vi "Parse.vi"(8 "Error In":errorcluster, 11 "Tokens":refnum<class "Abstract.lvclass">[](array[class])) -> (0 "Error Out":errorcluster, 3 "Abstract Syntax Tree":refnum<class "Root.lvclass">)   [LabVIEW 2018, in "Toolkit.lvlib"]
uses:
  Toolkit.lvlib
  Nodes/Root/Root.lvclass
  D:/Users/cfield/Code/Field R&D Services/Mustache/trunk/src/Toolkit/Low-Level/Nodes/NonTerminal/NonTerminal.lvclass
  Tokens/Abstract/Abstract.lvclass
  Nodes/NonTerminal/NonTerminal.lvclass
  D:/Users/cfield/Code/Field R&D Services/Mustache/trunk/src/Toolkit/Low-Level/Nodes/Abstract/Abstract.lvclass
  Tokens/Text/Text.lvclass
  Nodes/Section/Section.lvclass
  Nodes/Tag/Tag.lvclass
  Nodes/Text/Text.lvclass
  Tokens/Text/API/Read Content.vi
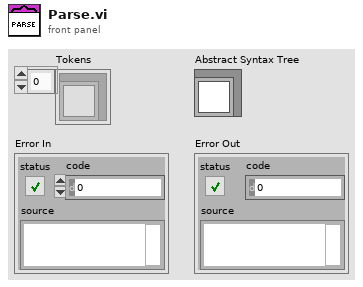
[diagram p1: front panel]
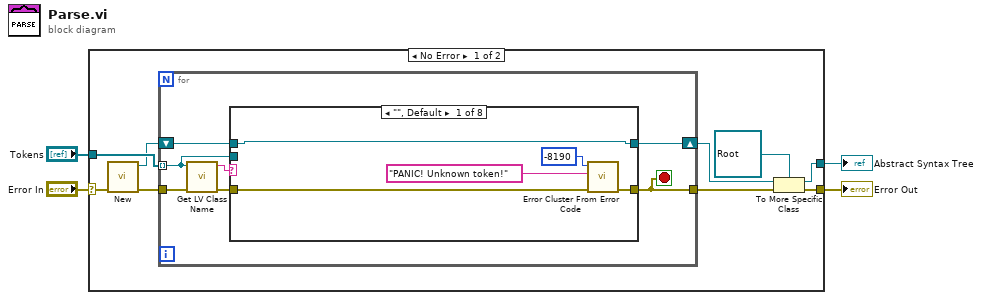
[diagram p0: block diagram]
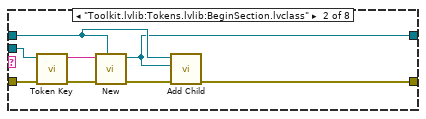
[diagram p2: hidden frame]
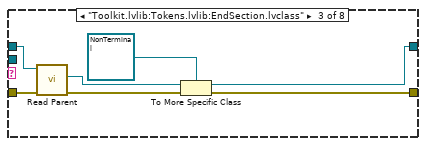
[diagram p3: hidden frame]
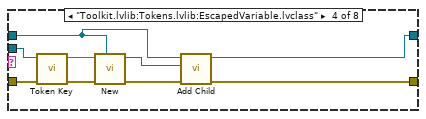
[diagram p4: hidden frame]
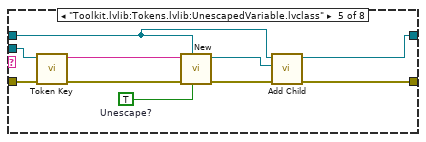
[diagram p5: hidden frame]
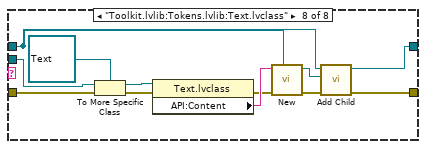
[diagram p8: hidden frame]
diagram:
  n1 = case shown="No Error" "Error In" {
    selector: "Error In" -> [w5 w76]
    tunnel: [w12 w76] -> w3
    tunnel: [w9 _] -> w2
    tunnel: "Tokens" -> [w8 _]
    frame No Error {
      n2 = call "New.vi"("Error In"=w5) -> ("Error Out"=w6:errorcluster, "Root"=w7:refnum<class "Root.lvclass">)  [unwired: 9 in]
      n3 = for {
        tunnel: w8 -> [w16] mode=indexing
        tunnel: w6 -> [w20]
        tunnel: [w17] -> w13
        shift-right: [w14] -> w11
        shift-left: w7 -> [w15]
        stop <- w17 stop-if-true
        n4 = call <vilib>:"Get LV Class Name.vi"("error in (no error)"=w20, "object"=w16) -> ("error out"=w18:errorcluster, "class name"=w19:string)  [unwired: 8 in]
        n5 = case shown="\"\", Default" w19 {
          tunnel: w18 -> [w25 w32 w38 w49 w53 w61 w63 w75]
          tunnel: [w23 w30 w37 w44 w56 w61 w63 w69] -> w17
          tunnel: w16 -> [_ w33 _ w48 w52 _ _ w73]
          tunnel: w15 -> [w21 w29 w40 w46 w58 w60 w62 w68]
          tunnel: [w21 w26 w34 w47 w59 w60 w62 w70] -> w14
          frame "", Default {
            n6 = call <vilib>:"Error Cluster From Error Code.vi"("error in (no error)"=w25, "error message (\"\")"="PANIC! Unknown token!" ("error message (\"\")"), "error code (0)"=-8190) -> ("error out"=w23:errorcluster)  [unwired: 6 in]
          }
          frame "Toolkit.lvlib:Tokens.lvlib:BeginSection.lvclass" {
            n7 = call "Token Key.vi"("Error In"=w32, "Token"=w33) -> ("Error Out"=w28:errorcluster, "Key"=w27:string)  [unwired: 8 in]
            n8 = call "New.vi"("Parent"=w29, "Error In"=w28, "Key"=w27) -> ("Error Out"=w31:errorcluster, "Section"=w26:refnum<class "Section.lvclass">)  [unwired: 7 in]
            n9 = call-dynamic "Add Child.vi"("Error In"=w31, "Child"=w26, "Non-Terminal In"=w29) -> ("Error Out"=w30:errorcluster)  [unwired: 7 in, 1 out]
          }
          frame "Toolkit.lvlib:Tokens.lvlib:EndSection.lvclass" {
            n10 = call-dynamic "Read Parent.vi"("Error In"=w38, "Abstract In"=w40) -> ("Error Out"=w39:errorcluster, "Parent"=w36:refnum<class "Abstract.lvclass">)  [unwired: 7 in, 1 out]
            n11 = To More Specific Class(target class=refnum<class "NonTerminal.lvclass"> refnum ("Toolkit.lvlib:Nodes.lvlib:NonTerminal.lvclass"), reference=w36, error in=w39) -> (specific class reference=w34:refnum<class "NonTerminal.lvclass">, error out=w37:errorcluster)
          }
          frame "Toolkit.lvlib:Tokens.lvlib:EscapedVariable.lvclass" {
            n12 = call "Token Key.vi"("Error In"=w49, "Token"=w48) -> ("Error Out"=w41:errorcluster, "Key"=w42:string)  [unwired: 8 in]
            n13 = call "New.vi"("Parent"=w46, "Error In"=w41, "Key"=w42) -> ("Error Out"=w45:errorcluster, "Tag"=w43:refnum<class "Tag.lvclass">)  [unwired: 7 in]
            n14 = call-dynamic "Add Child.vi"("Error In"=w45, "Child"=w43, "Non-Terminal In"=w46) -> ("Error Out"=w44:errorcluster, "Non-Terminal Out"=w47:refnum<class "NonTerminal.lvclass">)  [unwired: 7 in]
          }
          frame "Toolkit.lvlib:Tokens.lvlib:UnescapedVariable.lvclass" {
            w54 = TRUE  # Unescape?
            n15 = call "Token Key.vi"("Error In"=w53, "Token"=w52) -> ("Error Out"=w50:errorcluster, "Key"=w51:string)  [unwired: 8 in]
            n16 = call "New.vi"("Unescape?"=w54, "Parent"=w58, "Error In"=w50, "Key"=w51) -> ("Error Out"=w57:errorcluster, "Tag"=w55:refnum<class "Tag.lvclass">)  [unwired: 6 in]
            n17 = call-dynamic "Add Child.vi"("Error In"=w57, "Child"=w55, "Non-Terminal In"=w58) -> ("Error Out"=w56:errorcluster, "Non-Terminal Out"=w59:refnum<class "NonTerminal.lvclass">)  [unwired: 7 in]
          }
          frame "Toolkit.lvlib:Tokens.lvlib:InvertedSection.lvclass" {
            # "#TODO Add implemetation"
          }
          frame "Toolkit.lvlib:Tokens.lvlib:Partial.lvclass" {
            # "#TODO Add implemetation"
          }
          frame "Toolkit.lvlib:Tokens.lvlib:Text.lvclass" {
            n18 = To More Specific Class(target class=refnum<class "Text.lvclass"> refnum ("Toolkit.lvlib:Tokens.lvlib:Text.lvclass"), reference=w73, error in=w75) -> (specific class reference=w72:refnum<class "Text.lvclass">, error out=w71:errorcluster)
            n19 = property class="Text.lvclass"(reference=w72, error in=w71) -> (error out=w66:errorcluster, "API:Content"=w67:string)  [unwired: 1 out]
            n20 = call "New.vi"("Parent"=w68, "Error In"=w66, "Content"=w67) -> ("Error Out"=w65:errorcluster, "Text"=w64:refnum<class "Text.lvclass">)  [unwired: 7 in]
            n21 = call-dynamic "Add Child.vi"("Error In"=w65, "Child"=w64, "Non-Terminal In"=w68) -> ("Error Out"=w69:errorcluster, "Non-Terminal Out"=w70:refnum<class "NonTerminal.lvclass">)  [unwired: 7 in]
          }
        }
      }
      n22 = To More Specific Class(target class=refnum<class "Root.lvclass"> refnum ("Toolkit.lvlib:Nodes.lvlib:Root.lvclass"), reference=w11, error in=w13) -> (specific class reference=w9:refnum<class "Root.lvclass">, error out=w12:errorcluster)
    }
    frame Error {
    }
  }
  "Error Out" <- w3
  "Abstract Syntax Tree" <- w2
